vi "AutoClimb.vi"(7 "ClimbLevel":enum16{"2", "3"}(ring), 8 "BackLowSensor":dbl, 9 "FrontLowSensor":dbl, 10 "BackClimbEncoder":dbl, 11 "FrontClimbEncoder":dbl) -> (0 "ActuateBackClimb":dbl, 1 "ActuateFrontClimb":dbl, 2 "DropWheel":bool, 3 "ClimbDrive":bool)   [LabVIEW 2018]
uses:
  <vilib>/Rock Robotics/WPI/Utilities/WPI_GetSetVariantRefNum.vi
  Globals.vi
  <vilib>/Rock Robotics/Network Tables/NT Write Boolean.vi
  <vilib>/Rock Robotics/Network Tables/NT Write Number.vi
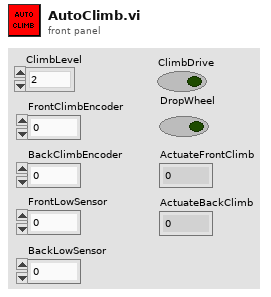
[diagram p1: front panel]
types:
  T1 = enum16{"initial climb", "elevated drive", "retract 1", "on platform drive", "retract 2", "finish"}
  T2 = typedef "WPI_CompressorDevRef.ctl" = cluster{"DevStatus":errorcluster, "Pneumatics Control Module":u8}
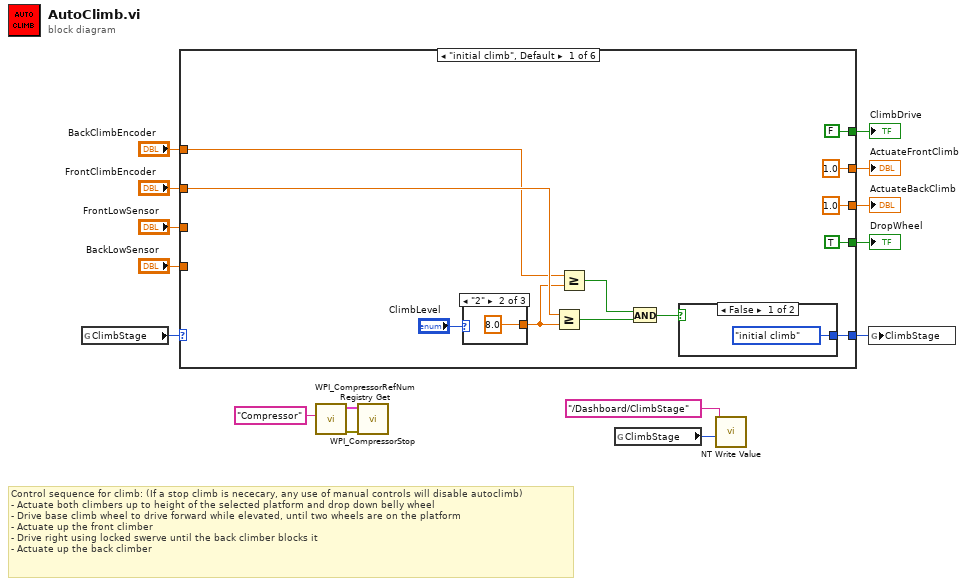
[diagram p0: block diagram]
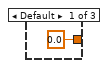
[diagram p2: hidden frame]
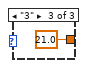
[diagram p3: hidden frame]
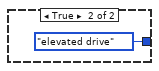
[diagram p4: hidden frame]
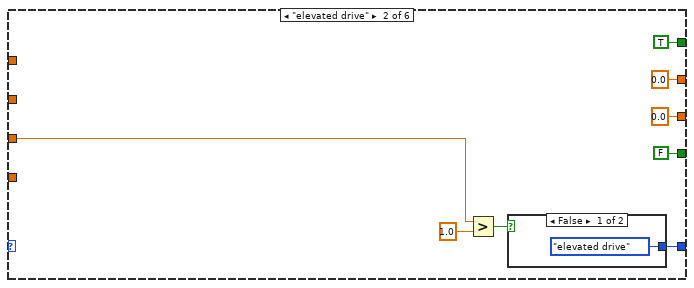
[diagram p5: hidden frame]
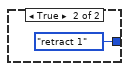
[diagram p6: hidden frame]
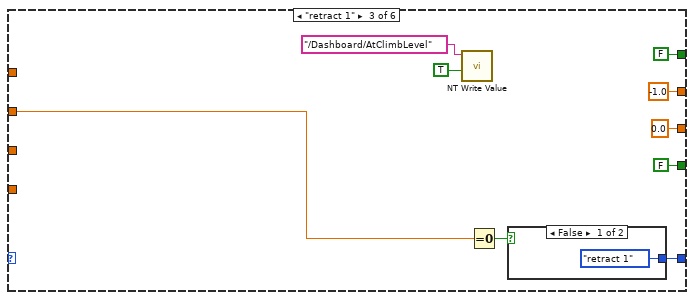
[diagram p7: hidden frame]
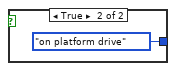
[diagram p8: hidden frame]
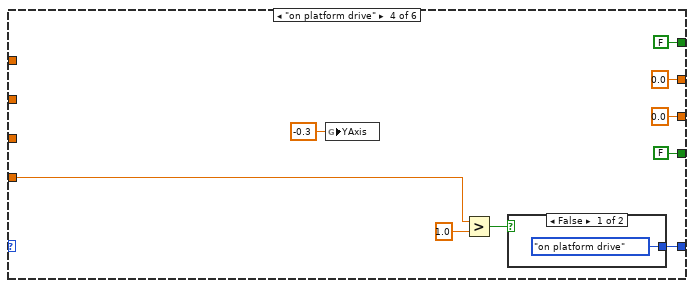
[diagram p9: hidden frame]
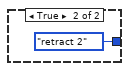
[diagram p10: hidden frame]
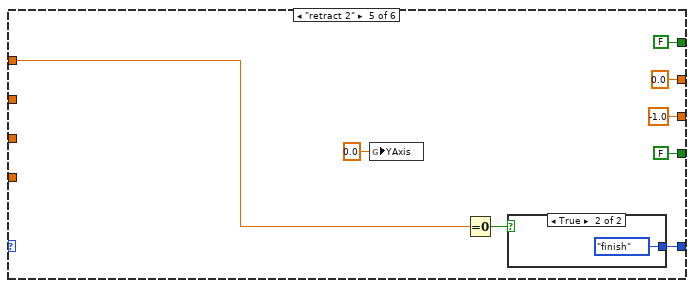
[diagram p11: hidden frame]
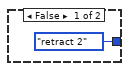
[diagram p12: hidden frame]
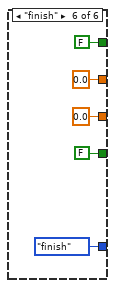
[diagram p13: hidden frame]
diagram:
  # "Control sequence for climb: (If a stop climb is nececary, any use of manual controls will disable autoclimb)\n- Actuate both climbers up to height of the selected platform and drop down belly wheel\n- Drive base climb wheel to drive forward while elevated, until two wheels are on the platform\n- Actuate up the front climber\n- Drive right using locked swerve until the back climber blocks it\n- Actuate up the back climber"
  n1 = global read "Globals.vi" "ClimbStage"() -> (w3:T1)
  n2 = case shown="\"initial climb\", Default" w3 {
    tunnel: [1.0 0.0 -1.0 0.0 0.0 0.0] -> w15
    tunnel: [1.0 0.0 0.0 0.0 -1.0 0.0] -> w14
    tunnel: [FALSE TRUE FALSE FALSE FALSE FALSE] -> w10
    tunnel: [TRUE FALSE FALSE FALSE FALSE FALSE] -> w9
    tunnel: "BackClimbEncoder" -> [w21 _ _ _ w71 _]
    tunnel: "FrontClimbEncoder" -> [w22 _ w46 _ _ _]
    tunnel: "FrontLowSensor" -> [_ w35 _ _ _ _]
    tunnel: "BackLowSensor" -> [_ _ _ w59 _ _]
    tunnel: [w24 w33 w51 w62 w72 T1."finish" ("Stage")] -> w4
    frame "initial climb", Default {
      n3 = case shown="\"2\"" "ClimbLevel" {
        tunnel: [0.0 8.0 21.0] -> w20
        frame Default {
        }
        frame "2" {
        }
        frame "3" {
        }
      }
      n4 = Greater Or Equal?(x=w22, y=w20) -> (x >= y?=w18:bool)
      n5 = Greater Or Equal?(x=w21, y=w20) -> (x >= y?=w19:bool)
      n6 = And(x=w19, y=w18) -> (x .and. y?=w17:bool)
      n7 = case shown="False" w17 {
        tunnel: [T1."initial climb" ("Stage") T1."elevated drive" ("Stage")] -> w24
        frame False {
        }
        frame True {
        }
      }
    }
    frame "elevated drive" {
      n8 = Greater?(x=w35, y=1.0) -> (0:w36:bool)
      n9 = case shown="False" w36 {
        tunnel: [T1."elevated drive" ("Stage") T1."retract 1" ("Stage")] -> w33
        frame False {
        }
        frame True {
        }
      }
    }
    frame "retract 1" {
      n10 = call-poly <vilib>:"NT Write Value.vi"("Boolean"=TRUE, "Name"="/Dashboard/AtClimbLevel") -> ()  [unwired: 9 in, 1 out]
      n11 = Equal To 0?(x=w46) -> (x = 0?=w45:bool)
      n12 = case shown="False" w45 {
        tunnel: [T1."retract 1" ("Stage") T1."on platform drive" ("Stage")] -> w51
        frame False {
        }
        frame True {
        }
      }
    }
    frame "on platform drive" {
      n13 = global write "Globals.vi" "YAxis"(-0.3 ("XAxis")) -> ()
      n14 = Greater?(x=w59, y=1.0) -> (0:w60:bool)
      n15 = case shown="False" w60 {
        tunnel: [T1."on platform drive" ("Stage") T1."retract 2" ("Stage")] -> w62
        frame False {
        }
        frame True {
        }
      }
    }
    frame "retract 2" {
      n16 = global write "Globals.vi" "YAxis"(0.0 ("XAxis")) -> ()
      n17 = Equal To 0?(x=w71) -> (x = 0?=w65:bool)
      n18 = case shown="True" w65 {
        tunnel: [T1."retract 2" ("Stage") T1."finish" ("Stage")] -> w72
        frame False {
        }
        frame True {
        }
      }
    }
    frame "finish" {
    }
  }
  "ActuateFrontClimb" <- w15
  "ClimbDrive" <- w10
  "ActuateBackClimb" <- w14
  "DropWheel" <- w9
  n19 = call <vilib>:"WPI_CompressorRefNum Registry Get.vi"("refnum name"="Compressor") -> ("error out"=w13:errorcluster, "CompressorDevRef"=w12:T2)  [unwired: 9 in]
  n20 = call <vilib>:"WPI_CompressorStop.vi"("error in (no error)"=w13, "CompressorDevRef"=w12) -> ()  [unwired: 8 in, 2 out]
  n21 = global read "Globals.vi" "ClimbStage"() -> (w1:T1)
  n22 = call-poly <vilib>:"NT Write Value.vi"("Numeric"=w1, "Name"="/Dashboard/ClimbStage") -> ()  [unwired: 9 in, 1 out]
  n23 = global write "Globals.vi" "ClimbStage"(w4) -> ()
